vi "DataLoggerScript.vi"() -> ()   [LabVIEW 2022 SP3]
uses:
  <vilib>/Utility/file.llb/Write Delimited Spreadsheet (DBL).vi
panel:
  in  "Save position data":bool
  out "Y Position record":dbl[](array[numeric])
  out "X Position record":dbl[](array[numeric])
  out "index":i32
  out "X Position record 2":dbl[](array[numeric])
  out "appended array":dbl[][](array[numeric])
  out "transposed array":dbl[][](array[numeric])
  out "Current position":dbl[](array[numeric]) format="%.6f"
  out "StageRunning":bool
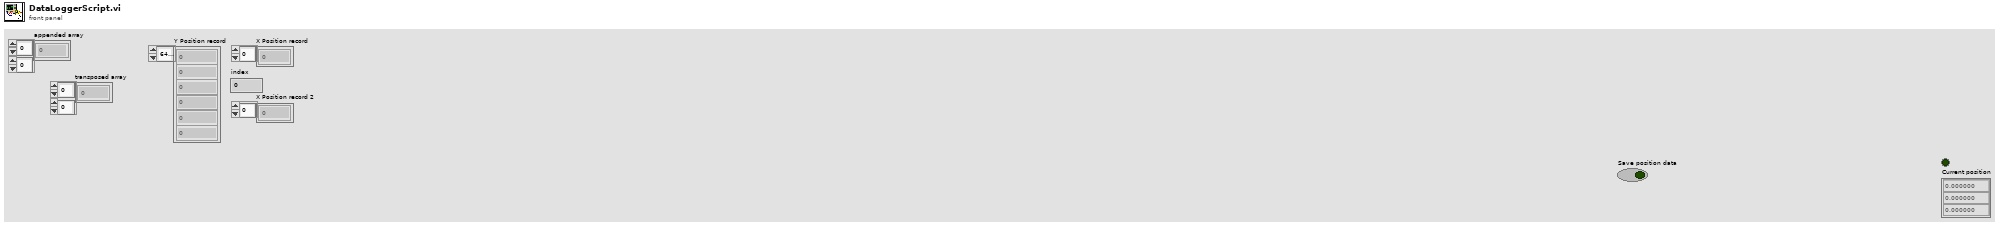
[diagram p1: front panel]
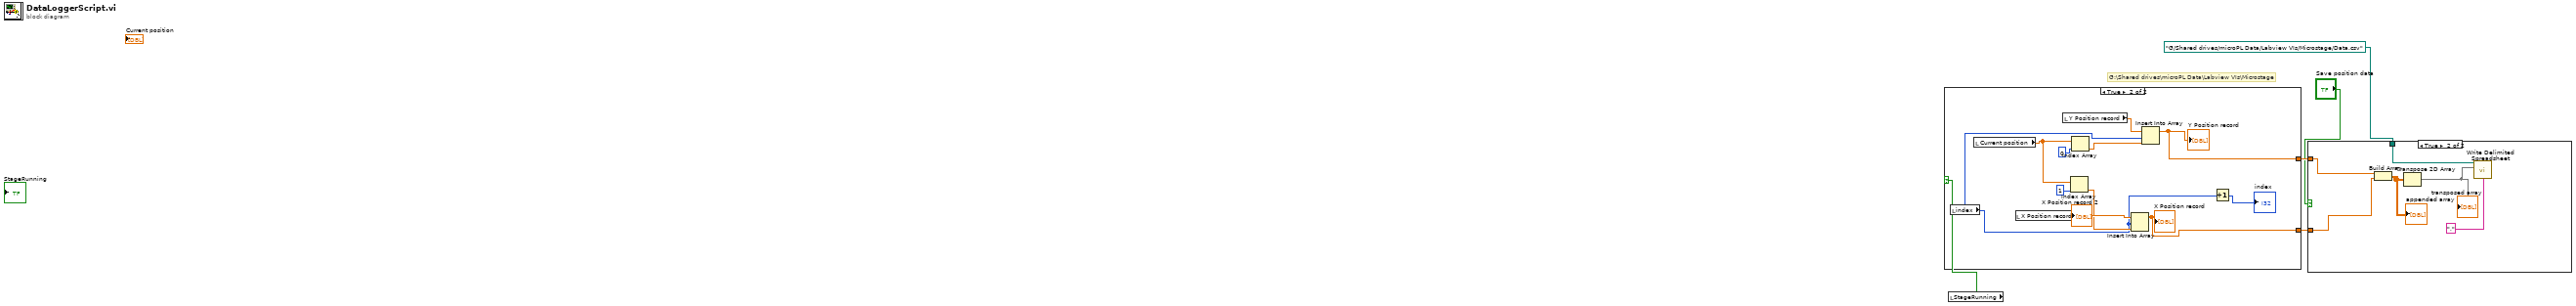
[diagram p0: block diagram]
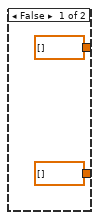
[diagram p2: hidden frame]
diagram:
  # "G:\\Shared drives\\microPL Data\\Labview VIs\\Microstage"
  n1 = local read "StageRunning"() -> (w2:bool)
  n2 = case shown="True" w2 {
    tunnel: [dbl[] [] ("Y Position record") w18] -> w5
    tunnel: [dbl[] [] ("X Position record") w17] -> w4
    frame False {
    }
    frame True {
      n3 = local read "index"() -> (w8:i32)
      n4 = local read "Current position"() -> (w11:dbl[])
      n5 = local read "X Position record"() -> (w16:dbl[])
      n6 = local read "Y Position record"() -> (w14:dbl[])
      n7 = Index Array(array=w11, index=1) -> (element=w15:dbl)
      n8 = Index Array(array=w11, index=0) -> (element=w10:dbl)
      n9 = Insert Into Array(array=w16, index=w8, new element=w15) -> (w17:dbl[])
      "X Position record" <- w17
      n10 = Insert Into Array(array=w14, index=w8, new element=w10) -> (w18:dbl[])
      "Y Position record" <- w18
      n11 = Increment(x=w8) -> (x+1=→"index":i32)
    }
  }
  n12 = case shown="True" "Save position data" {
    tunnel: w5 -> [_ w19]
    tunnel: w4 -> [_ w20]
    tunnel: path "G:/Shared drives/microPL Data/Labview VIs/Microstage/Data.csv" ("file path (dialog if empty)") -> [_ w23]
    frame False {
    }
    frame True {
      n13 = Build Array(w19, w20) -> (w22:dbl[][])
      "appended array" <- w22
      n14 = Transpose 2D Array(2D array=w22) -> (transposed array=w21:dbl[][])
      "transposed array" <- w21
      n15 = call-poly <vilib>:"Write Delimited Spreadsheet.vi"("file path (dialog if empty)"=w23, "2D data"=w21, "delimiter (\\t)"="," ("delimiter (\\t)")) -> ()  [unwired: 11 in, 2 out]
    }
  }
